vi "CD Init_Prepare Inline Data_Complete Broadcast Frame Descriptors.vi"(8 "error in (no error)":errorcluster, 10 "Broadcast Frame Descriptors In":T9[](array[typedef]) {"RTs"."Status Channel Ref" format="%.0x"; "RTs"."Words Block Data Refs"."Data Reference" format="%.0x"; "RTs"."Timestamp Channel Data Reference" format="%.0x"; "BC"."Status Channel Refs" format="%.0x"; "BC"."Words Block Data Refs"."Data Reference" format="%.0x"; "BC"."Timestamp Channel Data Reference" format="%.0x"}, 11 "RTs In":T1[](array[typedef]) {"Mode Codes"."Words Item Refs" format="%.0x"; "Mode Codes"."Words Block Data Refs"."Data Reference" format="%.0x"; "Mode Codes"."Timestamp Channel Data Reference" format="%.0x"; "subAddresses"."Words Item Refs" format="%.0x"; "subAddresses"."Words Block Data Refs"."Data Reference" format="%.0x"; "subAddresses"."Timestamp Channel Data Reference" format="%.0x"; "Status Channel Data Reference" format="%.0x"; "Command Channels Refs" format="%.0x"}) -> (0 "error out":errorcluster, 3 "Broadcast Frame Descriptors Out":T9[](array[typedef]) {"RTs"."Status Channel Ref" format="%.0x"; "RTs"."Words Block Data Refs"."Data Reference" format="%.0x"; "RTs"."Timestamp Channel Data Reference" format="%.0x"; "BC"."Status Channel Refs" format="%.0x"; "BC"."Words Block Data Refs"."Data Reference" format="%.0x"; "BC"."Timestamp Channel Data Reference" format="%.0x"})   [LabVIEW 2017, in "Ballard MIL-1553 Engine.lvlib"]
doc: "We complete Broadcast Frame Descriptors for frames not defined in BC (or there is no BC)."
uses:
  Ballard MIL-1553 Engine.lvlib
  Controls/RT Inline Broadcast Frame Descriptor.ctl
  Controls/RT Inline Frame Descriptor_BC.ctl
  <vilib>/NI Veristand/Custom Device API/Data Reference.ctl
  <vilib>/NI Veristand/Custom Device API/Block Data Reference.ctl
  <vilib>/NI Veristand/Custom Device API/Custom Device Item Ref.ctl
  Shared/Controls and Global/RT CWD2.ctl
  Shared/Controls and Global/RT CWD1.ctl
  Shared/Controls and Global/RT messageType.ctl
  Controls/RT Inline Frame Descriptor_RT.ctl
  Shared/Controls and Global/RT Remote Terminal.ctl
  Shared/Controls and Global/RT Remote Terminal_rtMode.ctl
  Shared/Controls and Global/RT Remote Terminal_RT subAddress.ctl
  Shared/Controls and Global/RT Remote Terminal_RT direction.ctl
  Shared/Controls and Global/RT Remote Terminal_RT Mode Code.ctl
  <vilib>/NI VeriStand/Custom Device Tools/Custom Device Utility Library/Custom Device Utility Library.lvlib
  Shared/Ballard 1553 Shared.lvlib
  <vilib>/NI VeriStand/Custom Device API/Custom Device API.lvlib
  Controls/RT Inline Frame Descriptor.ctl
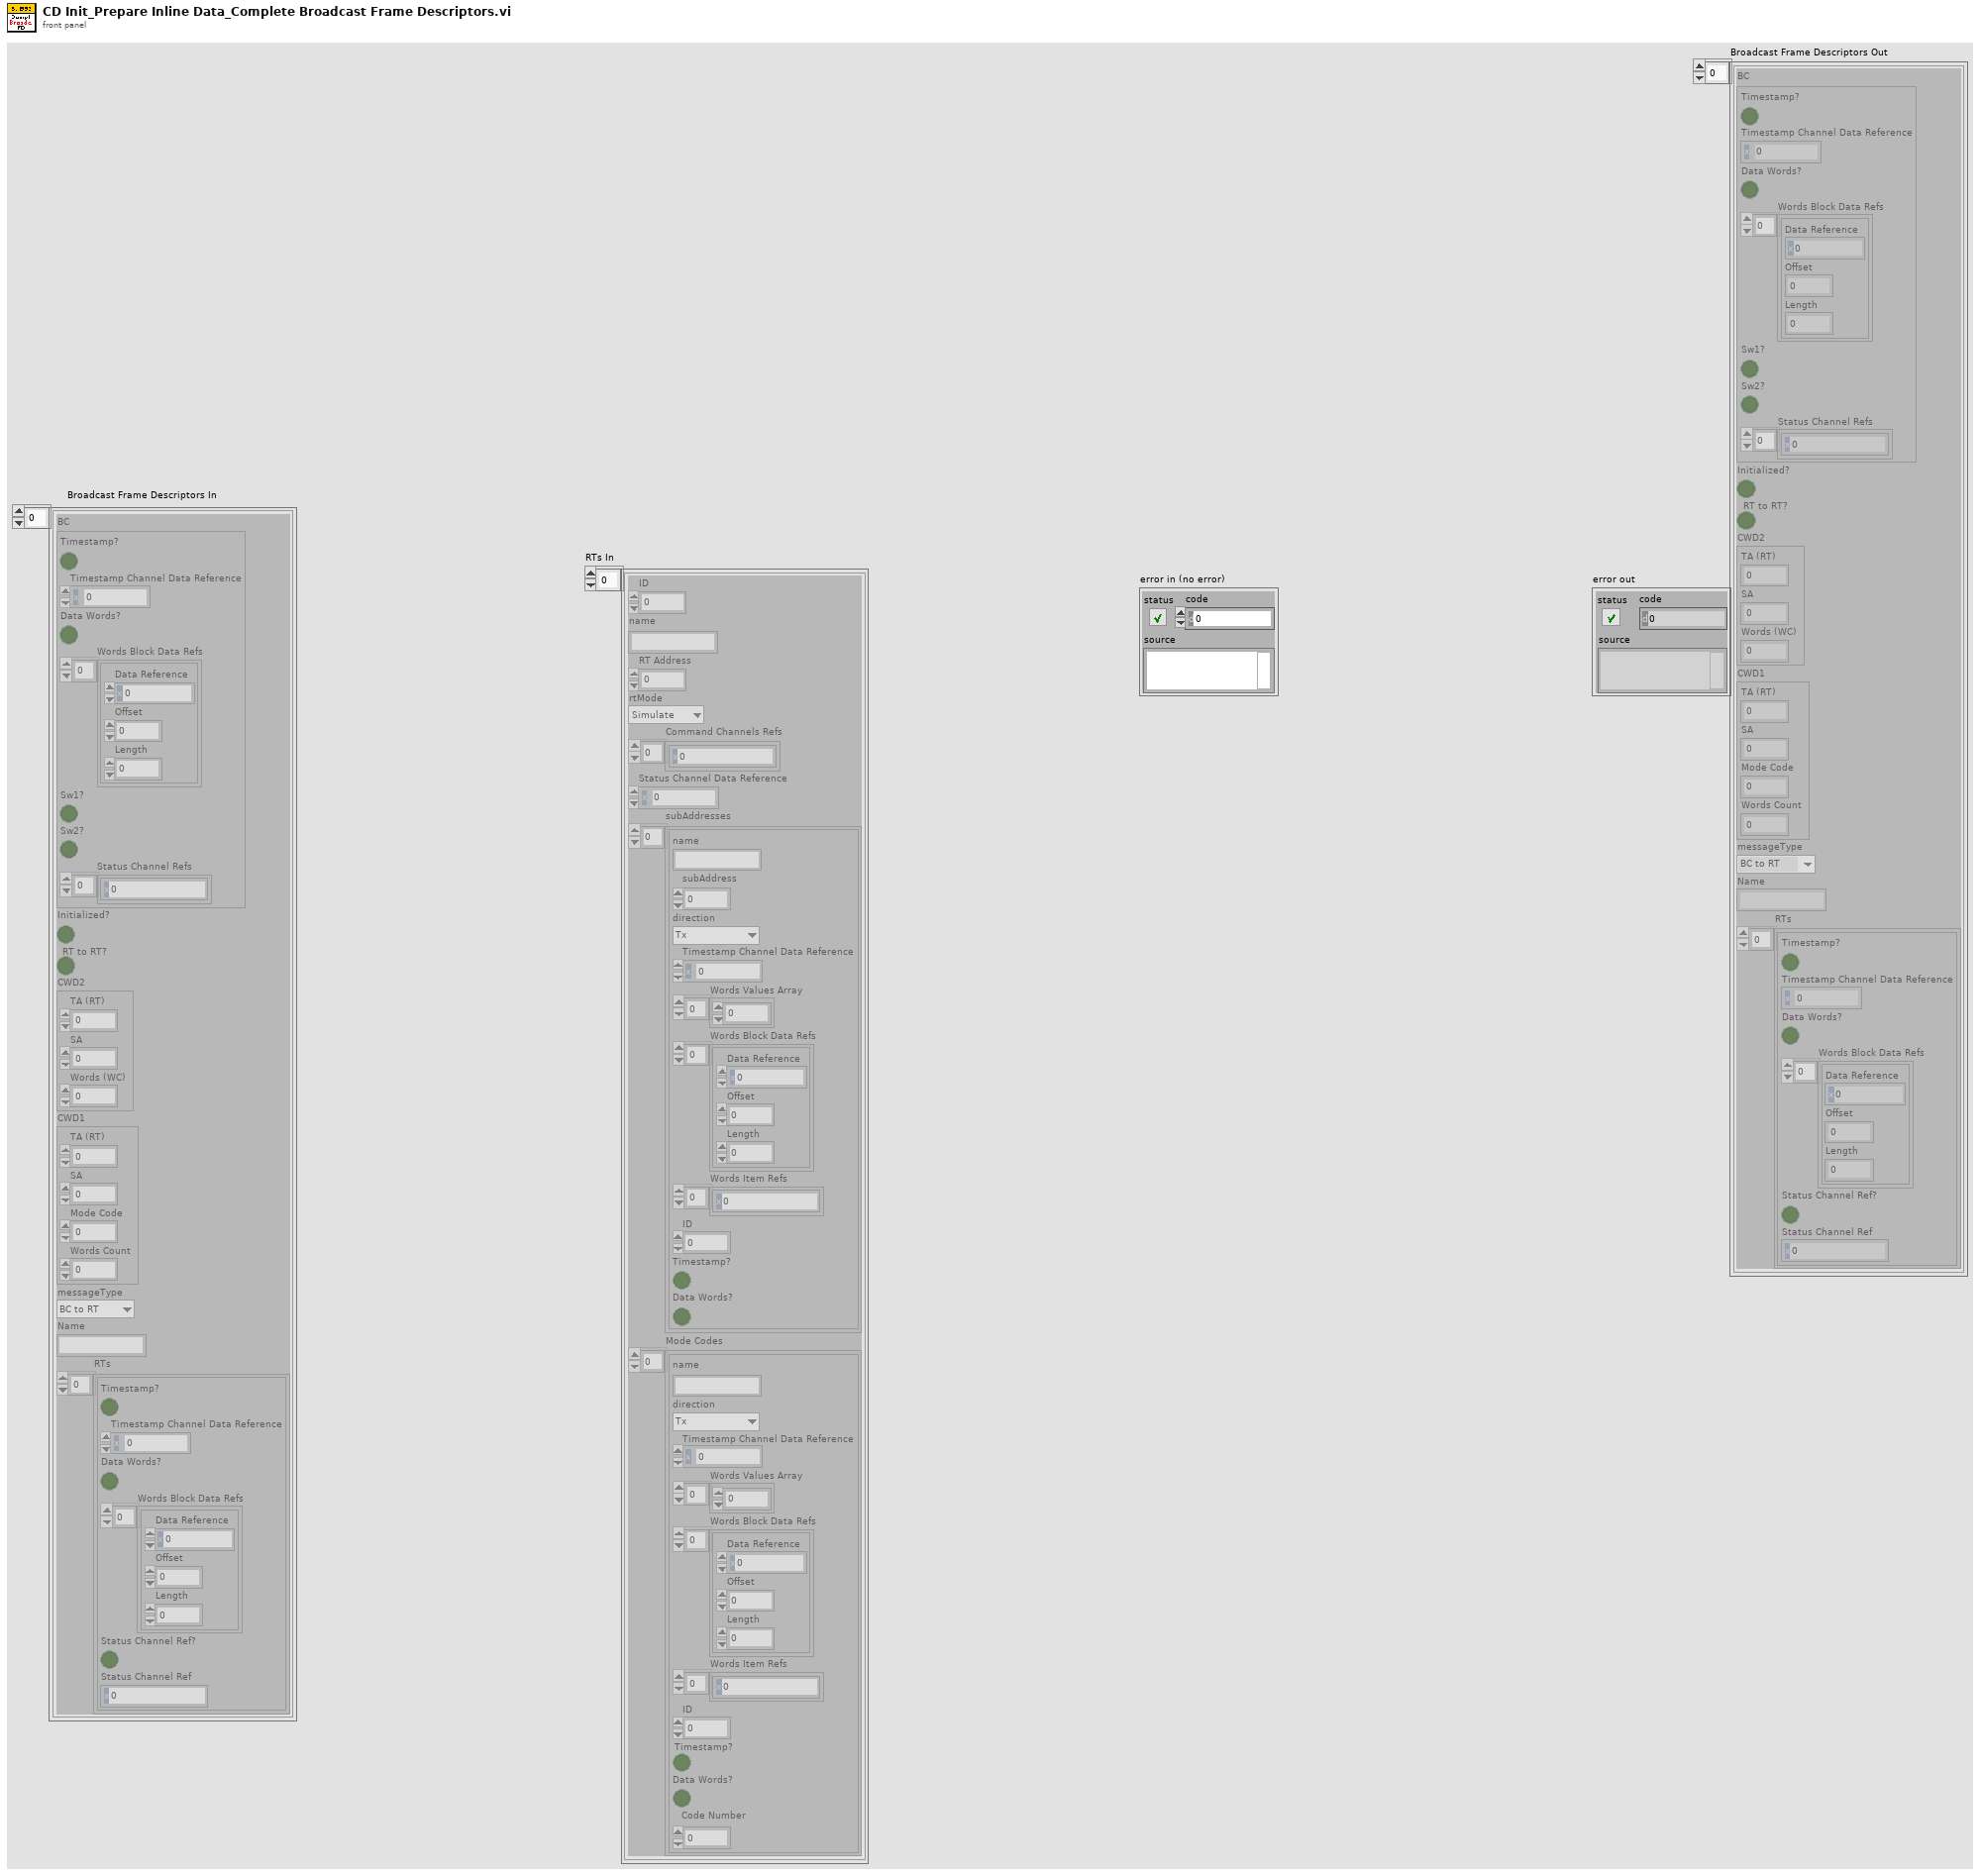
[diagram p1: front panel]
types:
  T1 = typedef "Ballard 1553 Shared.lvlib/RT Remote Terminal.ctl" = cluster{"ID":i32, "name":string, "RT Address":i32, "rtMode":T2, "Command Channels Refs":T3[], "Status Channel Data Reference":T4, "subAddresses":T5[], "Mode Codes":T8[]}
  T2 = typedef "Ballard 1553 Shared.lvlib/RT Remote Terminal_rtMode.ctl" = enum16{"Simulate", "Monitor", "Disable"}
  T3 = typedef "Custom Device API.lvlib/Custom Device Item Ref.ctl" = u64
  T4 = typedef "Custom Device API.lvlib/Data Reference.ctl" = i32
  T5 = typedef "Ballard 1553 Shared.lvlib/RT Remote Terminal_RT subAddress.ctl" = cluster{"name":string, "subAddress":i8, "direction":T6, "Timestamp Channel Data Reference":T4, "Words Values Array":u16[], "Words Block Data Refs":T7[], "Words Item Refs":T3[], "ID":i32, "Timestamp?":bool, "Data Words?":bool}
  T6 = typedef "Ballard 1553 Shared.lvlib/RT Remote Terminal_RT direction.ctl" = enum16{"Tx", "Rx"}
  T7 = typedef "Custom Device API.lvlib/Block Data Reference.ctl" = cluster{"Data Reference":T4, "Offset":u64, "Length":u64}
  T8 = typedef "Ballard 1553 Shared.lvlib/RT Remote Terminal_RT Mode Code.ctl" = cluster{"name":string, "direction":T6, "Timestamp Channel Data Reference":T4, "Words Values Array":u16[], "Words Block Data Refs":T7[], "Words Item Refs":T3[], "ID":i32, "Timestamp?":bool, "Data Words?":bool, "Code Number":i32}
  T9 = typedef "Ballard MIL-1553 Engine.lvlib/RT Inline Broadcast Frame Descriptor.ctl" = cluster{"BC":T10, "Initialized?":bool, "RT to RT?":bool, "CWD2":T11, "CWD1":T12, "messageType":T13, "Name":string, "RTs":T14[]}
  T10 = typedef "Ballard MIL-1553 Engine.lvlib/RT Inline Frame Descriptor_BC.ctl" = cluster{"Timestamp?":bool, "Timestamp Channel Data Reference":T4, "Data Words?":bool, "Words Block Data Refs":T7[], "Sw1?":bool, "Sw2?":bool, "Status Channel Refs":T3[]}
  T11 = typedef "Ballard 1553 Shared.lvlib/RT CWD2.ctl" = cluster{"TA (RT)":i8, "SA":i8, "Words (WC)":i8}
  T12 = typedef "Ballard 1553 Shared.lvlib/RT CWD1.ctl" = cluster{"TA (RT)":i8, "SA":i8, "Mode Code":i8, "Words Count":i8}
  T13 = typedef "Ballard 1553 Shared.lvlib/RT messageType.ctl" = enum16{"BC to RT", "RT to BC", "RT to RT", "MC (Rx)", "MC (Tx)"}
  T14 = typedef "Ballard MIL-1553 Engine.lvlib/RT Inline Frame Descriptor_RT.ctl" = cluster{"Timestamp?":bool, "Timestamp Channel Data Reference":T4, "Data Words?":bool, "Words Block Data Refs":T7[], "Status Channel Ref?":bool, "Status Channel Ref":T3}
  T15 = typedef "Ballard MIL-1553 Engine.lvlib/RT Inline Frame Descriptor.ctl" = cluster{"BC":T10, "RT":T14, "Initialized?":bool, "RT to RT?":bool, "CWD2":T11, "CWD1":T12, "messageType":T13, "Name":string}
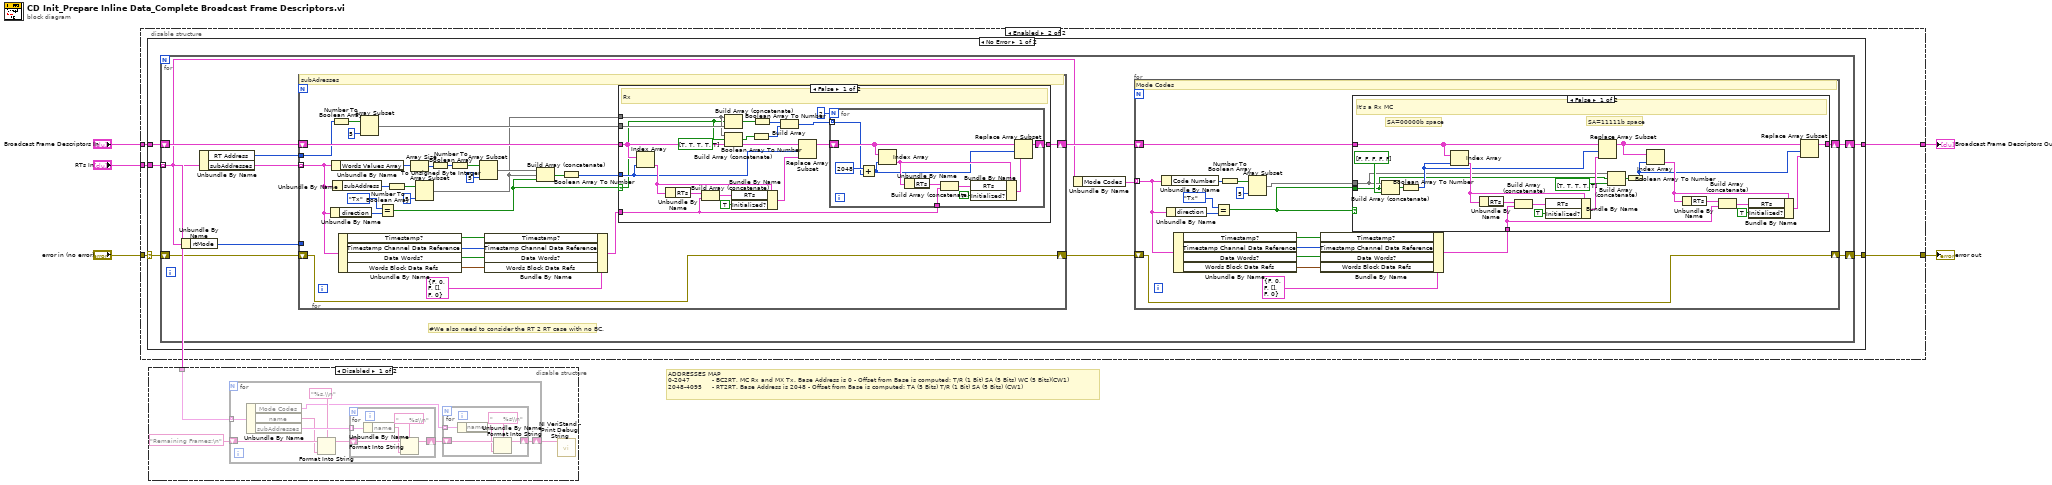
[diagram p0: block diagram]
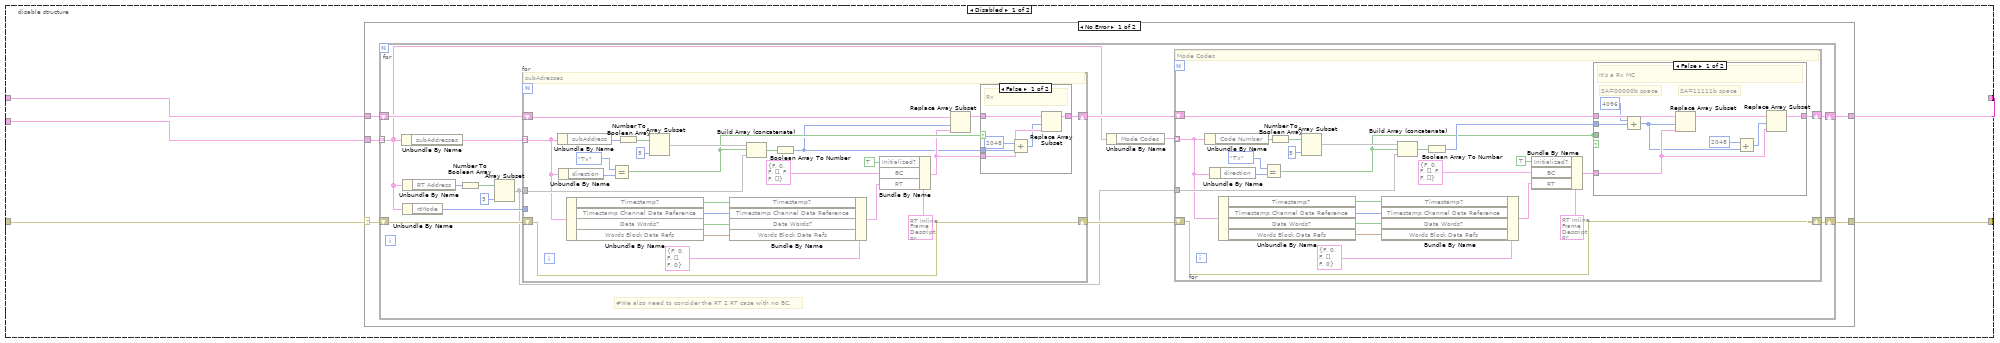
[diagram p2: hidden frame]
diagram:
  # "ADDRESSES MAP \n0-2047           - BC2RT, MC Rx and MX Tx. Base Address is 0 - Offset from Base is computed: T/R (1 Bit) SA (5 Bits) WC (5 Bits)(CW1)\n2048-4095     - RT2RT. Base Address is 2048 - Offset from Base is computed: TA (5 Bits) T/R (1 Bit) SA (5 Bits) (CW1)"
  n1 = disable-structure shown="Enabled" {
    disable-tunnel: [w10 w102] -> w5
    disable-tunnel: "error in (no error)" -> [w9 w101]
    disable-tunnel: "Broadcast Frame Descriptors In" -> [w8 w100]
    disable-tunnel: [w7 w99] -> w2
    disable-tunnel: "RTs In" -> [w6 w98]
    frame Disabled {
      n2 = case shown="No Error" w9 {
        selector: w9 -> [w11 w97]
        tunnel: [w15 w96] -> w7
        tunnel: w8 -> [w14 w96]
        tunnel: [w13 w97] -> w10
        tunnel: w6 -> [w12 _]
        frame No Error {
          n3 = for {
            tunnel: w12 -> [w18] mode=indexing
            shift-right: [w21] -> w15
            shift-left: w14 -> [w26]
            shift-right: [w19] -> w13
            shift-left: w11 -> [w23]
            # "#We also need to consider the RT 2 RT case with no BC."
            n4 = Unbundle By Name(w18) -> ("subAddresses"=w25:T5[])
            n5 = Unbundle By Name(w18) -> ("RT Address"=w27:i32)
            n6 = Unbundle By Name(w18) -> ("rtMode"=w24:T2)
            n7 = Number To Boolean Array(number=w27) -> (Boolean array=w28:bool[])
            n8 = Array Subset(array=w28, length=5) -> (w16:bool[])  [unwired: 1 in]
            n9 = for {
              tunnel: w16 -> [w81]
              shift-right: [w68] -> w22
              shift-left: w26 -> [w80]
              tunnel: w25 -> [w75] mode=indexing
              tunnel: w24 -> [_]
              shift-right: [w64] -> w20
              shift-left: w23 -> [w64]
              # "subAdresses"
              n10 = Unbundle By Name(w75) -> ("subAddress"=w86:i8)
              n11 = Unbundle By Name(w75) -> ("direction"=w83:T6)
              n12 = Unbundle By Name(w75) -> ("Timestamp?"=w74:bool, "Timestamp Channel Data Reference"=w72:T4, "Data Words?"=w71:bool, "Words Block Data Refs"=w70:T7[])
              n13 = Equal?(x=RT_Remote_Terminal_RT_direction."Tx", y=w83) -> (x = y?=w67:bool)
              n14 = Number To Boolean Array(number=w86) -> (Boolean array=w87:bool[])
              n15 = Array Subset(array=w87, length=5) -> (w84:bool[])  [unwired: 1 in]
              n16 = Bundle By Name(cluster=T14 {"Timestamp?"=FALSE, "Timestamp Channel Data Reference"=0, "Data Words?"=FALSE, "Words Block Data Refs"=[], "Status Channel Ref?"=FALSE, "Status Channel Ref"=0} ("RT"), "Timestamp?"=w74, "Timestamp Channel Data Reference"=w72, "Data Words?"=w71, "Words Block Data Refs"=w70) -> (w73:T14)
              n17 = Build Array (concatenate)(w84, w67, w81) -> (w85:bool[])
              n18 = Boolean Array To Number(Boolean array=w85) -> (number=w65:u16)
              n19 = Bundle By Name(cluster=T15 {"BC"={"Timestamp?"=FALSE, "Timestamp Channel Data Reference"=0, "Data Words?"=FALSE, "Words Block Data Refs"=[], "Sw1?"=FALSE, "Sw2?"=FALSE, "Status Channel Refs"=[]}, "RT"={"Timestamp?"=FALSE, "Timestamp Channel Data Reference"=0, "Data Words?"=FALSE, "Words Block Data Refs"=[], "Status Channel Ref?"=FALSE, "Status Channel Ref"=0}, "Initialized?"=FALSE, "RT to RT?"=FALSE, "CWD2"={"TA (RT)"=0, "SA"=0, "Words (WC)"=0}, "CWD1"={"TA (RT)"=0, "SA"=0, "Mode Code"=0, "Words Count"=0}, "messageType"=enum."BC to RT", "Name"=""} ("Frame Descriptor"), "Initialized?"=TRUE, "BC"=T10 {"Timestamp?"=FALSE, "Timestamp Channel Data Reference"=0, "Data Words?"=FALSE, "Words Block Data Refs"=[], "Sw1?"=FALSE, "Sw2?"=FALSE, "Status Channel Refs"=[]}, "RT"=w73) -> (w66:T15)
              n20 = Replace Array Subset(array=w80, new element=w66, index=w65) -> (w69:T9[])
              n21 = case shown="False" w67 {
                tunnel: w69 -> [w94 w95]
                tunnel: [w93 w95] -> w68
                tunnel: w66 -> [w92 _]
                tunnel: w65 -> [w91 _]
                frame False {
                  # "Rx"
                  n22 = Add(x=u16 2048, y=w91) -> (x+y=w90:u16)
                  n23 = Replace Array Subset(array=w94, new element=w92, index=w90) -> (w93:T9[])
                }
                frame True {
                }
              }
            }
            n24 = Unbundle By Name(w18) -> ("Mode Codes"=w17:T8[])
            n25 = for {
              tunnel: w16 -> [w46]
              shift-right: [w34] -> w21
              shift-left: w22 -> [w45]
              tunnel: w17 -> [w40] mode=indexing
              shift-right: [w31] -> w19
              shift-left: w20 -> [w31]
              # "Mode Codes"
              n26 = Unbundle By Name(w40) -> ("Code Number"=w51:i32)
              n27 = Unbundle By Name(w40) -> ("direction"=w48:T6)
              n28 = Unbundle By Name(w40) -> ("Timestamp?"=w39:bool, "Timestamp Channel Data Reference"=w37:T4, "Data Words?"=w36:bool, "Words Block Data Refs"=w35:T7[])
              n29 = Equal?(x=RT_Remote_Terminal_RT_direction."Tx", y=w48) -> (x = y?=w30:bool)
              n30 = Number To Boolean Array(number=w51) -> (Boolean array=w52:bool[])
              n31 = Array Subset(array=w52, length=5) -> (w49:bool[])  [unwired: 1 in]
              n32 = Bundle By Name(cluster=T14 {"Timestamp?"=FALSE, "Timestamp Channel Data Reference"=0, "Data Words?"=FALSE, "Words Block Data Refs"=[], "Status Channel Ref?"=FALSE, "Status Channel Ref"=0} ("RT"), "Timestamp?"=w39, "Timestamp Channel Data Reference"=w37, "Data Words?"=w36, "Words Block Data Refs"=w35) -> (w38:T14)
              n33 = Build Array (concatenate)(w49, w30, w46) -> (w50:bool[])
              n34 = Boolean Array To Number(Boolean array=w50) -> (number=w32:u16)
              n35 = Bundle By Name(cluster=T15 {"BC"={"Timestamp?"=FALSE, "Timestamp Channel Data Reference"=0, "Data Words?"=FALSE, "Words Block Data Refs"=[], "Sw1?"=FALSE, "Sw2?"=FALSE, "Status Channel Refs"=[]}, "RT"={"Timestamp?"=FALSE, "Timestamp Channel Data Reference"=0, "Data Words?"=FALSE, "Words Block Data Refs"=[], "Status Channel Ref?"=FALSE, "Status Channel Ref"=0}, "Initialized?"=FALSE, "RT to RT?"=FALSE, "CWD2"={"TA (RT)"=0, "SA"=0, "Words (WC)"=0}, "CWD1"={"TA (RT)"=0, "SA"=0, "Mode Code"=0, "Words Count"=0}, "messageType"=enum."BC to RT", "Name"=""} ("Frame Descriptor"), "Initialized?"=TRUE, "BC"=T10 {"Timestamp?"=FALSE, "Timestamp Channel Data Reference"=0, "Data Words?"=FALSE, "Words Block Data Refs"=[], "Sw1?"=FALSE, "Sw2?"=FALSE, "Status Channel Refs"=[]}, "RT"=w38) -> (w33:T15)
              n36 = case shown="False" w30 {
                tunnel: w45 -> [w62 w63]
                tunnel: [w60 w63] -> w34
                tunnel: w30 -> [_ _]
                tunnel: w33 -> [w59 _]
                tunnel: w32 -> [w58 _]
                frame False {
                  # "SA=11111b space"
                  # "SA=00000b space"
                  # "It's a Rx MC"
                  n37 = Add(x=u16 4096, y=w58) -> (x+y=w57:u16)
                  n38 = Replace Array Subset(array=w62, new element=w59, index=w57) -> (w61:T9[])
                  n39 = Add(x=u16 2048, y=w57) -> (x+y=w55:u16)
                  n40 = Replace Array Subset(array=w61, new element=w59, index=w55) -> (w60:T9[])
                }
                frame True {
                  # "Tx"
                }
              }
            }
          }
        }
        frame Error {
        }
      }
    }
    frame Enabled {
      n41 = case shown="No Error" w101 {
        selector: w101 -> [w103 w221]
        tunnel: [w107 w220] -> w99
        tunnel: w100 -> [w106 w220]
        tunnel: [w105 w221] -> w102
        tunnel: w98 -> [w104 _]
        frame No Error {
          n42 = for {
            tunnel: w104 -> [w110] mode=indexing
            shift-right: [w113] -> w107
            shift-left: w106 -> [w118]
            shift-right: [w111] -> w105
            shift-left: w103 -> [w115]
            # "#We also need to consider the RT 2 RT case with no BC."
            n43 = Unbundle By Name(w110) -> ("rtMode"=w116:T2)
            n44 = Unbundle By Name(w110) -> ("RT Address"=w108:i32, "subAddresses"=w117:T5[])
            n45 = for {
              shift-right: [w176] -> w114
              shift-left: w118 -> [w165]
              tunnel: w117 -> [w174] mode=indexing
              tunnel: w116 -> [_]
              shift-right: [w175] -> w112
              shift-left: w115 -> [w175]
              tunnel: w108 -> [w161]
              # "subAdresses"
              n46 = Unbundle By Name(w174) -> ("direction"=w183:T6)
              n47 = Unbundle By Name(w174) -> ("Words Values Array"=w173:u16[])
              n48 = Number To Boolean Array(number=w161) -> (Boolean array=w163:bool[])
              n49 = Unbundle By Name(w174) -> ("subAddress"=w185:i8)
              n50 = Unbundle By Name(w174) -> ("Timestamp?"=w180:bool, "Timestamp Channel Data Reference"=w179:T4, "Data Words?"=w178:bool, "Words Block Data Refs"=w177:T7[])
              n51 = Array Subset(array=w163, length=5) -> (w160:bool[])  [unwired: 1 in]
              n52 = Equal?(x=RT_Remote_Terminal_RT_direction."Tx", y=w183) -> (x = y?=w166:bool)
              n53 = Number To Boolean Array(number=w185) -> (Boolean array=w186:bool[])
              n54 = Array Size(array=w173) -> (size(s)=w172:i32)
              n55 = Array Subset(array=w186, length=5) -> (w159:bool[])  [unwired: 1 in]
              n56 = To Unsigned Byte Integer(number=w172) -> (unsigned 8bit integer=w169:u8)
              n57 = Number To Boolean Array(number=w169) -> (Boolean array=w171:bool[])
              n58 = Array Subset(array=w171, length=5) -> (w168:bool[])  [unwired: 1 in]
              n59 = Bundle By Name(cluster=T14 {"Timestamp?"=FALSE, "Timestamp Channel Data Reference"=0, "Data Words?"=FALSE, "Words Block Data Refs"=[], "Status Channel Ref?"=FALSE, "Status Channel Ref"=0} ("RT"), "Timestamp?"=w180, "Timestamp Channel Data Reference"=w179, "Data Words?"=w178, "Words Block Data Refs"=w177) -> (w167:T14)
              n60 = Build Array (concatenate)(w168, w159, w166) -> (w184:bool[])
              n61 = Boolean Array To Number(Boolean array=w184) -> (number=w164:u16)
              n62 = case shown="False" w166 {
                selector: w166 -> [w189 _]
                tunnel: w165 -> [w201 w219]
                tunnel: [w207 w219] -> w176
                tunnel: w164 -> [w199 _]
                tunnel: w167 -> [w198 _]
                tunnel: w160 -> [w197 _]
                tunnel: w159 -> [w190 _]
                frame False {
                  # "Rx"
                  n63 = Index Array(array=w201, index=w199) -> (element=w206:T9)
                  n64 = Unbundle By Name(w206) -> ("RTs"=w205:T14[])
                  n65 = Build Array (concatenate)(w205, w198) -> (w204:T14[])
                  n66 = Build Array (concatenate)(w190, w189, w197) -> (w193:bool[])
                  n67 = Build Array (concatenate)(w190, w189, bool[] [TRUE, TRUE, TRUE, TRUE, TRUE]) -> (w192:bool[])
                  n68 = Bundle By Name(cluster=w206, "RTs"=w204, "Initialized?"=TRUE) -> (w203:T9)
                  n69 = Boolean Array To Number(Boolean array=w192) -> (number=w191:u16)
                  n70 = Boolean Array To Number(Boolean array=w193) -> (number=w195:u16)
                  n71 = Build Array(w195, w191) -> (w194:u16[])
                  n72 = Replace Array Subset(array=w201, new element=w203, index=w199) -> (w200:T9[])
                  n73 = for {
                    N: 2 -> [_]
                    tunnel: w198 -> [w209]
                    tunnel: w194 -> [w208] mode=indexing
                    shift-right: [w218] -> w207
                    shift-left: w200 -> [w210]
                    n74 = Add(x=u16 2048, y=w208) -> (x+y=w212:u16)
                    n75 = Index Array(array=w210, index=w212) -> (element=w213:T9)
                    n76 = Unbundle By Name(w213) -> ("RTs"=w214:T14[])
                    n77 = Build Array (concatenate)(w214, w209) -> (w215:T14[])
                    n78 = Bundle By Name(cluster=w213, "RTs"=w215, "Initialized?"=TRUE) -> (w211:T9)
                    n79 = Replace Array Subset(array=w210, new element=w211, index=w212) -> (w218:T9[])
                  }
                }
                frame True {
                }
              }
            }
            n80 = Unbundle By Name(w110) -> ("Mode Codes"=w109:T8[])
            n81 = for {
              shift-right: [w123] -> w113
              shift-left: w114 -> [w130]
              tunnel: w109 -> [w128] mode=indexing
              shift-right: [w122] -> w111
              shift-left: w112 -> [w122]
              # "Mode Codes"
              n82 = Unbundle By Name(w128) -> ("Code Number"=w133:i32)
              n83 = Unbundle By Name(w128) -> ("direction"=w132:T6)
              n84 = Unbundle By Name(w128) -> ("Timestamp?"=w127:bool, "Timestamp Channel Data Reference"=w126:T4, "Data Words?"=w125:bool, "Words Block Data Refs"=w124:T7[])
              n85 = Equal?(x=RT_Remote_Terminal_RT_direction."Tx", y=w132) -> (x = y?=w120:bool)
              n86 = Number To Boolean Array(number=w133) -> (Boolean array=w134:bool[])
              n87 = Array Subset(array=w134, length=5) -> (w121:bool[])  [unwired: 1 in]
              n88 = Bundle By Name(cluster=T14 {"Timestamp?"=FALSE, "Timestamp Channel Data Reference"=0, "Data Words?"=FALSE, "Words Block Data Refs"=[], "Status Channel Ref?"=FALSE, "Status Channel Ref"=0} ("RT"), "Timestamp?"=w127, "Timestamp Channel Data Reference"=w126, "Data Words?"=w125, "Words Block Data Refs"=w124) -> (w119:T14)
              n89 = case shown="False" w120 {
                tunnel: w130 -> [w155 w158]
                tunnel: [w157 w158] -> w123
                tunnel: w121 -> [w146 _]
                tunnel: w120 -> [w145 _]
                tunnel: w119 -> [w139 _]
                frame False {
                  # "SA=11111b space"
                  # "SA=00000b space"
                  # "It's a Rx MC"
                  n90 = Build Array (concatenate)(w146, w145, bool[] [FALSE, FALSE, FALSE, FALSE, FALSE]) -> (w156:bool[])
                  n91 = Boolean Array To Number(Boolean array=w156) -> (number=w149:u16)
                  n92 = Index Array(array=w155, index=w149) -> (element=w151:T9)
                  n93 = Unbundle By Name(w151) -> ("RTs"=w154:T14[])
                  n94 = Build Array (concatenate)(w154, w139) -> (w153:T14[])
                  n95 = Bundle By Name(cluster=w151, "RTs"=w153, "Initialized?"=TRUE) -> (w150:T9)
                  n96 = Replace Array Subset(array=w155, new element=w150, index=w149) -> (w147:T9[])
                  n97 = Build Array (concatenate)(w146, w145, bool[] [TRUE, TRUE, TRUE, TRUE, TRUE]) -> (w143:bool[])
                  n98 = Boolean Array To Number(Boolean array=w143) -> (number=w137:u16)
                  n99 = Index Array(array=w147, index=w137) -> (element=w138:T9)
                  n100 = Unbundle By Name(w138) -> ("RTs"=w140:T14[])
                  n101 = Build Array (concatenate)(w140, w139) -> (w141:T14[])
                  n102 = Bundle By Name(cluster=w138, "RTs"=w141, "Initialized?"=TRUE) -> (w136:T9)
                  n103 = Replace Array Subset(array=w147, new element=w136, index=w137) -> (w157:T9[])
                }
                frame True {
                  # "Tx"
                }
              }
            }
          }
        }
        frame Error {
        }
      }
    }
  }
  "error out" <- w5
  "Broadcast Frame Descriptors Out" <- w2
  n104 = disable-structure shown="Disabled" {
    disable-tunnel: "RTs In" -> [w224 _]
    frame Disabled {
      n105 = for {
        tunnel: w224 -> [w233] mode=indexing
        shift-right: [w227] -> w222
        shift-left: "Remaining Frames:\n" -> [w231]
        n106 = Unbundle By Name(w233) -> ("Mode Codes"=w225:T8[], "name"=w230:string, "subAddresses"=w232:T5[])
        n107 = Format Into String(format string="%s,\\n", initial string=w231, w230) -> (resulting string=w228:string)  [unwired: 1 in, 1 out]
        n108 = for {
          tunnel: w232 -> [w243] mode=indexing
          shift-right: [w242] -> w226
          shift-left: w228 -> [w241]
          n109 = Unbundle By Name(w243) -> ("name"=w240:string)
          n110 = Format Into String(format string="     %s\\n", initial string=w241, w240) -> (resulting string=w242:string)  [unwired: 1 in, 1 out]
        }
        n111 = for {
          tunnel: w225 -> [w238] mode=indexing
          shift-right: [w237] -> w227
          shift-left: w226 -> [w236]
          n112 = Unbundle By Name(w238) -> ("name"=w235:string)
          n113 = Format Into String(format string="     %s\\n", initial string=w236, w235) -> (resulting string=w237:string)  [unwired: 1 in, 1 out]
        }
      }
      n114 = call <vilib>:"NI VeriStand - Print Debug String.vi"("Message"=w222) -> ()  [unwired: 10 in, 1 out]
    }
    frame Enabled {
    }
  }
